vi "GetMessageFile.vi"(3 "type":string) -> (0 "error out":errorcluster, 1 "File":string)   [LabVIEW 2012]
doc: "Returns ROS message file"
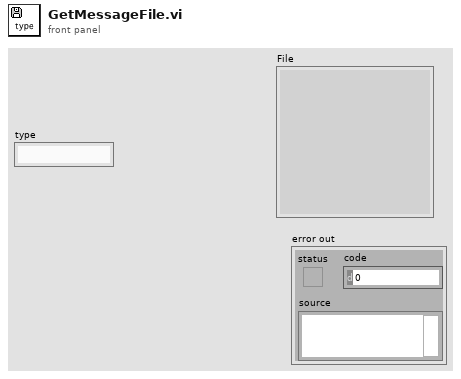
[diagram p1: front panel]
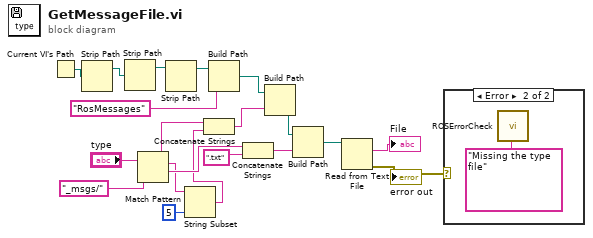
[diagram p0: block diagram]
diagram:
  n1 = Current VI's Path() -> (path=w16:path)
  n2 = Strip Path(path=w16) -> (stripped path=w12:path)  [unwired: 1 out]
  n3 = Strip Path(path=w12) -> (stripped path=w11:path)  [unwired: 1 out]
  n4 = Match Pattern(string="type", regular expression="_msgs/" ("search string")) -> (before substring=w5:string, match substring=w3:string, after substring=w6:string)  [unwired: 1 in, 1 out]
  n5 = Strip Path(path=w11) -> (stripped path=w13:path)  [unwired: 1 out]
  n6 = String Subset(string=w3, length (rest)=5 ("length (rest)")) -> (substring=w2:string)  [unwired: 1 in]
  n7 = Concatenate Strings(w5, w2) -> (w4:string)
  n8 = Build Path(base path=w13, name or relative path="RosMessages" ("string")) -> (appended path=w10:path)
  n9 = Concatenate Strings(w6, ".txt" ("string")) -> (w20:string)
  n10 = Build Path(base path=w10, name or relative path=w4) -> (appended path=w9:path)
  n11 = Build Path(base path=w9, name or relative path=w20) -> (appended path=w17:path)
  n12 = Read from Text File(file (use dialog)=w17) -> (text=→"File":string, error out=w14:errorcluster)  [unwired: 3 in, 2 out]
  "error out" <- w14
  n13 = case shown="Error" w14 {
    frame No Error {
    }
    frame Error {
      n14 = call <userlib>:"ROSErrorCheck.vi"("message"="Missing the type file") -> ()  [unwired: 2 in, 1 out]
    }
  }
